vi "Spring Analysis.vi"() -> ()   [LabVIEW 2024]
uses:
  <vilib>/Utility/file.llb/Read Delimited Spreadsheet (DBL).vi
  <vilib>/gmath/NI_Gmath.lvlib
  <vilib>/Analysis/NI_AALPro.lvlib
panel:
  in  "Skip points (raw data)":i32
  out "Spectrum":T1(graph)=[{"time start"=0.0, "df"=0.49751243781094523, "Power Spectrum (V^2 rms)"=[5.644866949331598e-05, 0.00013686624305728217, 0.00022038571008669523, 0.00041028831547446017, 0.0008486507694054388, 0.002042096260864871, 0.006435671488207052, 0.020896992615224798, 0.010543505206445309, 0.00392758055394729, 0.001991571736893036, 0.0012169525544927543, 0.0008310812614828688, 0.0006098344085945337, 0.0004702652862590481, 0.000375985799513062, 0.0003089575120970624, 0.00025938177290646495, 0.00022154504395459433, 0.00019192243396481184, 0.00016823708014891692, 0.00014896115841386858, 0.00013303604254786888, 0.00011970786081307353, 0.00010842694010669756, 9.878417014082367e-05, 9.046951026584988e-05, 8.324421425577846e-05, 7.692180036901625e-05, 7.135474003886612e-05, 6.642497195524682e-05, 6.203702789756774e-05, 5.811297495461124e-05, 5.45886423520356e-05, 5.1410770806166024e-05, 4.853483372999109e-05, 4.5923354075646326e-05, 4.35445911853837e-05, 4.1371506917581324e-05, 3.938094472334656e-05, 3.7552972647060335e-05, 3.5870353631410695e-05, 3.431811550787647e-05, 3.288319965156931e-05, 3.155417216432179e-05, 3.032098510000748e-05, 2.917477799758377e-05, 2.8107712078341994e-05, 2.7112831065381034e-05, 2.6183943818827068e-05, 2.531552494024343e-05, 2.4502630250260028e-05, 2.3740824634033174e-05, 2.3026120216663534e-05, 2.235492320285061e-05, 2.1723988012796467e-05, 2.1130377585996665e-05, 2.0571428918158274e-05, 2.00447230537285e-05, 1.9548058884826993e-05, 1.9079430212451e-05, 1.8637005612268403e-05, 1.821911071872427e-05, 1.782421260036284e-05, 1.745090594850682e-05, 1.709790084256156e-05, 1.676401188963703e-05, 1.644814856514056e-05, 1.614930660539041e-05, 1.586656032393563e-05, 1.559905574077967e-05, 1.5346004428575323e-05, 1.5106677992571845e-05, 1.4880403111937629e-05, 1.4666557079393808e-05, 1.4464563784095495e-05, 1.4273890089585874e-05, 1.4094042564606332e-05, 1.392456452969376e-05, 1.3765033386971049e-05, 1.361505820442835e-05, 1.347427752938351e-05, 1.33423574087637e-05, 1.3218989596459617e-05, 1.3103889930277334e-05, 1.299679686299879e-05, 1.2897470133867677e-05, 1.2805689568343873e-05, 1.2721253995378978e-05, 1.2643980272694602e-05, 1.2573702411648248e-05, 1.2510270794245523e-05, 1.2453551475767183e-05, 1.2403425567259563e-05, 1.235978869287705e-05, 1.2322550517711422e-05, 1.2291634342378541e-05, 1.2266976761162613e-05, 1.224852738106678e-05, 1.2236248599588424e-05]}, {"time start"=0.0, "df"=0.5, "Power Spectrum (V^2 rms)"=[5.6303024605838505e-05, 0.00013698521619382454, 0.00022207111065130337, 0.0004162057648891435, 0.0008670327309824444, 0.002106953935671304, 0.006743647337272303, 0.02134435548843732, 0.010152944032489135, 0.003818664652887894, 0.0019521631638462402, 0.0011987461426457172, 0.000821227351523806, 0.0006039020886803867, 0.00046641372855931893, 0.00037334112300694406, 0.0003070617209886131, 0.00025797588434058424, 0.0002204735430536851, 0.00019108728072320526, 0.00016757393291649876, 0.00014842634075070798, 0.00013259904044947505, 0.00011934682035404783, 0.00010812586743173314, 9.853113532263249e-05, 9.02554633827969e-05, 8.306218604029104e-05, 7.676635083863324e-05, 7.122157081563383e-05, 6.63106489246679e-05, 6.193877966903397e-05, 5.802854430021882e-05, 5.451617525819134e-05, 5.134873261558307e-05, 4.8481945054995685e-05, 4.587854131814135e-05, 4.3506947970481254e-05, 4.1340263767530726e-05, 3.935544501430629e-05, 3.753265340009534e-05, 3.585473005500931e-05, 3.430676847514845e-05, 3.287576549051895e-05, 3.155033428420553e-05, 3.0320467084980642e-05, 2.9177337880358707e-05, 2.8113137568557535e-05, 2.7120935554807088e-05, 2.6194563022143593e-05, 2.5328514058508867e-05, 2.4517861566365142e-05, 2.375818546688881e-05, 2.3045511174664717e-05, 2.2376256688083065e-05, 2.1747186936257198e-05, 2.1155374261103743e-05, 2.059816410551022e-05, 2.0073145134689127e-05, 1.9578123145254e-05, 1.9111098220952924e-05, 1.8670244679907133e-05, 1.8253893429150234e-05, 1.7860516401094542e-05, 1.7488712795505423e-05, 1.713719689143336e-05, 1.680478722781218e-05, 1.6490396980207004e-05, 1.6193025385476953e-05, 1.5911750086642064e-05, 1.5645720287655987e-05, 1.5394150622599654e-05, 1.5156315656440666e-05, 1.4931544945310561e-05, 1.471921859351259e-05, 1.451876325243961e-05, 1.432964851343845e-05, 1.4151383652589758e-05, 1.3983514690501608e-05, 1.3825621734668978e-05, 1.3677316575829607e-05, 1.353824051312092e-05, 1.3408062385798106e-05, 1.3286476791860006e-05, 1.3173202476199866e-05, 1.3067980872899705e-05, 1.2970574788048847e-05, 1.2880767211031191e-05, 1.2798360243613115e-05, 1.2723174137392796e-05, 1.2655046431280431e-05, 1.2593831181663405e-05, 1.2539398278799699e-05, 1.249163284378996e-05, 1.2450434701207355e-05, 1.2415717923134284e-05, 1.2387410440970289e-05, 1.2365453721942524e-05, 1.234980250778595e-05, 1.2340424613557116e-05]}]
  out "w_n":dbl=22.360679774997898
  out "lambda":dbl=2.5
  out "phi":dbl=-6.379370208442803
  out "zeta":dbl=0.11180339887498948
  out "w":dbl=22.22048604328897
  in  "h (step rate)":dbl=0.01 format="%#_13g"
  in  "time end":dbl=2.0 format="%#_13g"
  out "formula":string="(1/0.2)*(0 - 100.0*x-1.0*v)"
  in  "b (kg/s)":dbl=1.0
  in  "k (N/m)":dbl=100.0
  in  "m (kg)":dbl=0.2
  out "XY Graph":cluster{"t":dbl[], "y":dbl[]}[](graph)=[{"t"=[0.0, 0.01, 0.02, 0.03, 0.04, 0.05, 0.06, 0.07, 0.08, 0.09, 0.1, 0.11, 0.12, 0.13, 0.14, 0.15, 0.16, 0.17, 0.18, 0.19, 0.2, 0.21, 0.22, 0.23, 0.24, 0.25, 0.26, 0.27, 0.28, 0.29, 0.3, 0.31, 0.32, 0.33, 0.34, 0.35000000000000003, 0.36, 0.37, 0.38, 0.39, 0.4, 0.41000000000000003, 0.42, 0.43, 0.44, 0.45, 0.46, 0.47000000000000003, 0.48, 0.49, 0.5, 0.51, 0.52, 0.53, 0.54, 0.55, 0.56, 0.5700000000000001, 0.58, 0.59, 0.6, 0.61, 0.62, 0.63, 0.64, 0.65, 0.66, 0.67, 0.68, 0.6900000000000001, 0.7000000000000001, 0.71, 0.72, 0.73, 0.74, 0.75, 0.76, 0.77, 0.78, 0.79, 0.8, 0.81, 0.8200000000000001, 0.8300000000000001, 0.84, 0.85, 0.86, 0.87, 0.88, 0.89, 0.9, 0.91, 0.92, 0.93, 0.9400000000000001, 0.9500000000000001, 0.96, 0.97, 0.98, 0.99, 1.0, 1.01, 1.02, 1.03, 1.04, 1.05, 1.06, 1.07, 1.08, 1.09, 1.1, 1.11, 1.12, 1.1300000000000001, 1.1400000000000001, 1.1500000000000001, 1.16, 1.17, 1.18, 1.19, 1.2, 1.21, 1.22, 1.23, 1.24, 1.25, 1.26, 1.27, 1.28, 1.29, 1.3, 1.31, 1.32, 1.33, 1.34, 1.35, 1.36, 1.37, 1.3800000000000001, 1.3900000000000001, 1.4000000000000001, 1.41, 1.42, 1.43, 1.44, 1.45, 1.46, 1.47, 1.48, 1.49, 1.5, 1.51, 1.52, 1.53, 1.54, 1.55, 1.56, 1.57, 1.58, 1.59, 1.6, 1.61, 1.62, 1.6300000000000001, 1.6400000000000001, 1.6500000000000001, 1.6600000000000001, 1.67, 1.68, 1.69, 1.7, 1.71, 1.72, 1.73, 1.74, 1.75, 1.76, 1.77, 1.78, 1.79, 1.8, 1.81, 1.82, 1.83, 1.84, 1.85, 1.86, 1.87, 1.8800000000000001, 1.8900000000000001, 1.9000000000000001, 1.9100000000000001, 1.92, 1.93, 1.94, 1.95, 1.96, 1.97, 1.98, 1.99, 2.0], "y"=[1.0, 0.975515625, 0.9048485799953885, 0.793683069664252, 0.6493929363281531, 0.4806011443268373, 0.29670008251256486, 0.10735789255481054, -0.07796451989619155, -0.2504628554170456, -0.40238498785058513, -0.5273561409768714, -0.6206213150931946, -0.6791972253554723, -0.7019307857362803, -0.6894658557932868, -0.6441243389898921, -0.569711583964797, -0.4712592311333951, -0.35472104410393157, -0.22663879090384154, -0.09379586235376258, 0.037123952080977934, 0.15985621065048394, 0.26883960656418304, 0.3594517673889705, 0.4281879550488793, 0.4727767722975505, 0.49223032830694485, 0.4868296232894181, 0.4580490211512866, 0.408426448734615, 0.3413882722918879, 0.26103956647665394, 0.1719316493186711, 0.07881928171138101, -0.01358017275140981, -0.10081402659302488, -0.1788976092955688, -0.2444849621427372, -0.29500018918659987, -0.32872500386549935, -0.34484035571892346, -0.34342235495225737, -0.3253949215470226, -0.292443568976384, -0.24689640504851432, -0.19157972789914587, -0.1296564691558737, -0.06445616690920357, 0.0006948609412173318, 0.06263490496802816, 0.11851238768904226, 0.16590922844963654, 0.20293713901309063, 0.22830349328088, 0.24134505591305894, 0.2420294992244689, 0.2309262055651196, 0.20914927105365919, 0.17827683439769085, 0.14025180322280553, 0.09726970640911173, 0.05165974680670299, 0.005765162700131027, -0.03817125792537532, -0.0781112015116528, -0.11230984961723836, -0.1393863044836639, -0.158372906037056, -0.16874207461187324, -0.1704104717672045, -0.16372138325677194, -0.1494072417839289, -0.1285350781827299, -0.10243838276656284, -0.07263934879204084, -0.04076574338519084, -0.008466705164658923, 0.022668389739429782, 0.0511842025707476, 0.07582357501558565, 0.09557891939612398, 0.10972898210465766, 0.1178599081398488, 0.11987034932104397, 0.1159611462422494, 0.10661083736652331, 0.09253887585301797, 0.07465893998148106, 0.054025087799386425, 0.03177372000252235, 0.009064374089703692, -0.012977717833028039, -0.03331460388033973, -0.05104176494358258, -0.0654255362421032, -0.07593040624916397, -0.08223536085077696, -0.08423901320416048, -0.08205381705083081, -0.07599017688950663, -0.06653171941364053, -0.05430335821716742, -0.04003405418447279, -0.024516338813351385, -0.008564724116440714, 0.007024926743547271, 0.021513141739166665, 0.03425000299447483, 0.04470234326186144, 0.05247394601235676, 0.05731810930030696, 0.05914233562598567, 0.05800530402270094, 0.0541066477962295, 0.04777038521758563, 0.039423117399039344, 0.02956830738133625, 0.018758080697674012, 0.007564037813668293, -0.0034514558511086115, -0.013762131287019213, -0.02290161425167547, -0.030483154208638476, -0.03621452415003514, -0.03990760318392188, -0.04148243580729574, -0.04096584007979952, -0.03848489812848742, -0.03425589469726605, -0.028569462935715474, -0.02177284379663645, -0.014250261390446144, -0.006402459262850092, 0.0013735676474944157, 0.008703670580218948, 0.015253603645054814, 0.02074331079027449, 0.024957884261405716, 0.02775482466611119, 0.02906743041485267, 0.028904340686160886, 0.02734544169485179, 0.0245345124303503, 0.020669126037913037, 0.01598843112513127, 0.010759509794696634, 0.005263044345776378, -0.00022097753341185095, -0.005426826720042466, -0.010115242655414573, -0.014083762428217628, -0.017174759029140417, -0.019280910109926268, -0.020347956959430813, -0.020374751853478153, -0.019410723717520652, -0.01755101108606643, -0.014929612490192732, -0.011710983614726916, -0.008080565062751212, -0.004234752905569823, -0.0003708262803258748, 0.003322676695688286, 0.006674689155693872, 0.00953907145920618, 0.011800492949357306, 0.01337853060978188, 0.014229872523405239, 0.014348611543999279, 0.013764708053206304, 0.012540785749171647, 0.010767497375390532, 0.008557755197001334, 0.006040161789274618, 0.0033519991759583434, 0.0006321383437194483, -0.001985782629107675, -0.004379593619351125, -0.006443966489134685, -0.008094709094618867, -0.009271823401027234, -0.0099412394552807, -0.010095205579256125, -0.009751381366060609, -0.008950740789438657, -0.007754445291027591, -0.006239888937871361, -0.004496148096187246, -0.0026190856517750516, -0.0007063643913824762, 0.0011473838458313055, 0.0028550062291457018, 0.004340696853274629, 0.005543124955016649, 0.0064177075783471696, 0.0069379580370410926, 0.007095889756472437, 0.006901501948259575, 0.006381416872882789]}, ...(2 in all)]
  # "Spring Mass Damper Model\n\nThis compares a Runga-Kutta solution to the analytical one.\n\nYou can add forcing if you want"
  # "Simulation parameters"
  # "Spring parameters"
  # "Calculated parameters"
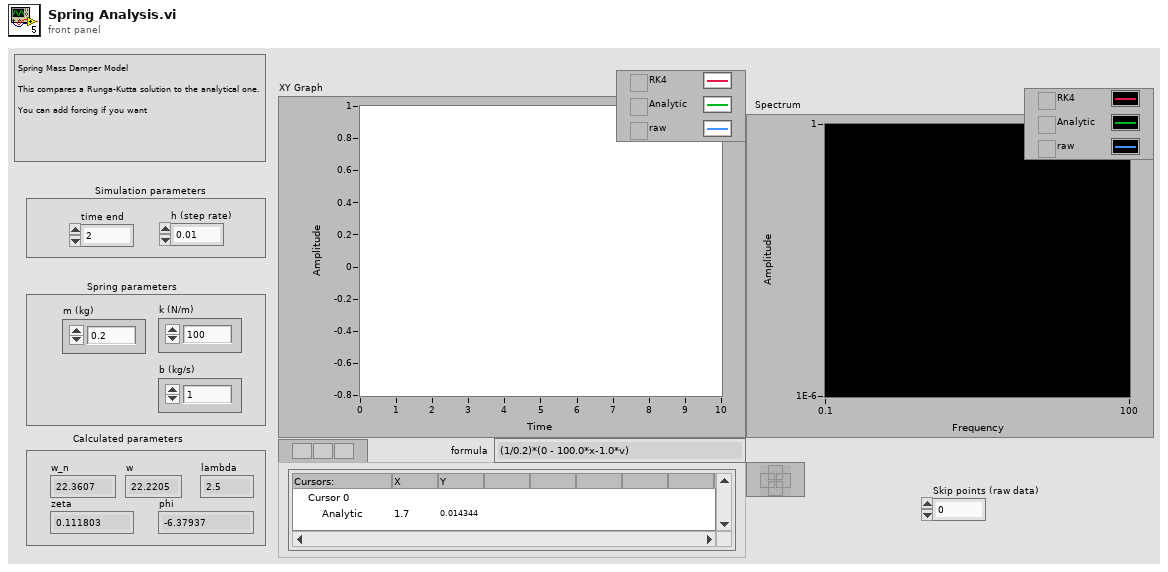
[diagram p1: front panel]
types:
  T1 = cluster{"time start":dbl, "df":dbl, "Power Spectrum (V^2 rms)":dbl[]}[]
  T2 = cluster{"time start":dbl, "df":dbl, "Power Spectrum (V^2 rms)":dbl[]}
  T3 = cluster{"Times":dbl[], "X Values (solution)":dbl[]}
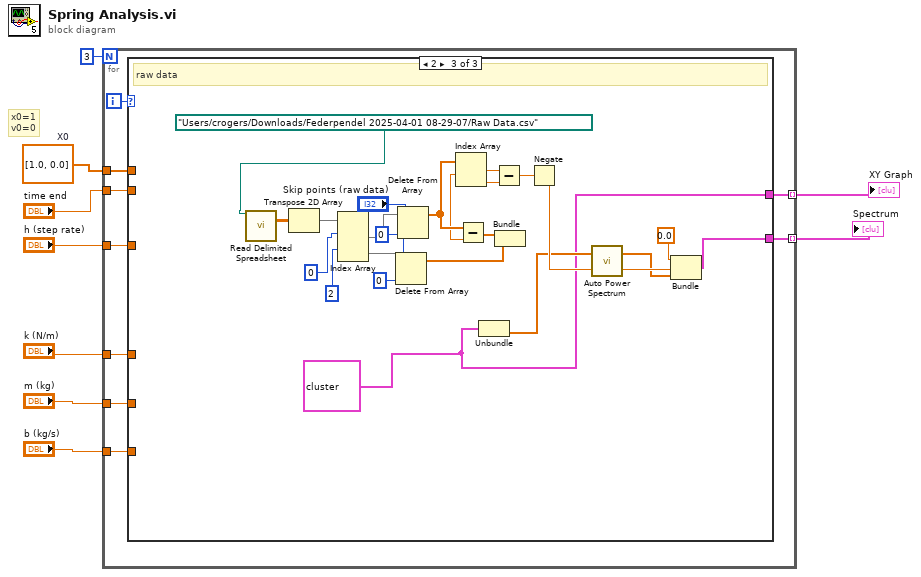
[diagram p0: block diagram]
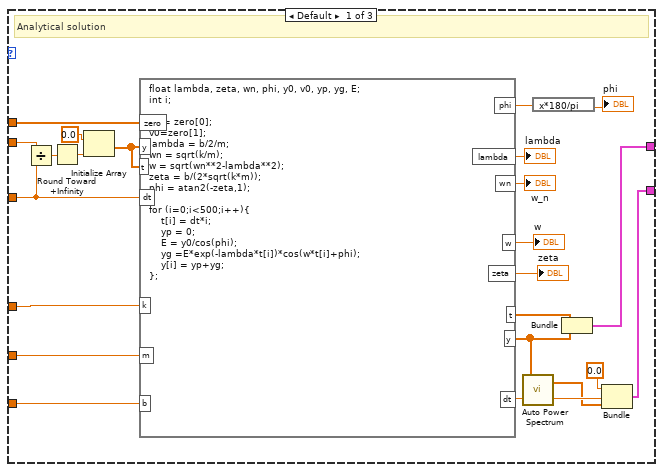
[diagram p2: hidden frame]
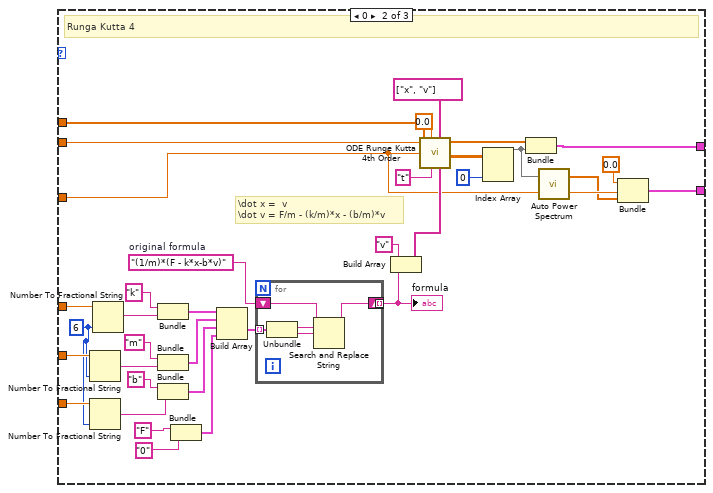
[diagram p3: hidden frame]
diagram:
  w5 = dbl[] [1.0, 0.0]  # X0
  # "x0=1\nv0=0"
  n1 = for {
    N: 3 -> [_]
    tunnel: "k (N/m)" -> [w18]
    tunnel: "m (kg)" -> [w17]
    tunnel: "b (kg/s)" -> [w16]
    tunnel: [w15] -> w4 mode=indexing
    tunnel: w5 -> [w14]
    tunnel: "h (step rate)" -> [w12]
    tunnel: "time end" -> [w11]
    tunnel: [w10] -> w1 mode=indexing
    i -> [w13]
    n2 = case shown="2" w13 {
      tunnel: w18 -> [w34 w61 _]
      tunnel: w17 -> [w33 w60 _]
      tunnel: w16 -> [w32 w59 _]
      tunnel: [w31 w58 w85] -> w15
      tunnel: w14 -> [w35 w57 _]
      tunnel: w12 -> [w29 w53 _]
      tunnel: w11 -> [w30 w56 _]
      tunnel: [w19 w49 w96] -> w10
      frame Default {
        # "Analytical solution"
        n3 = Divide(x=w30, y=w29) -> (x/y=w28:dbl)
        n4 = Round Toward +Infinity(x=w28) -> (ceil(x): smallest int >= x=w27:dbl)
        n5 = Initialize Array(0.0 ("element"), w27) -> (w39:dbl[])
        n6 = formula code="float lambda, zeta, wn, phi, y0, v0, yp, yg, E;\nint i;\n\ny0 = zero[0];\nv0=zero[1];\nlambda = b/2/m;\nwn = sqrt(k/m);\nw = sqrt(wn**2-lambda**2);\nzeta = b/(2*sqrt(k*m));\nphi = atan2(-zeta,1);\n\nfor (i=0;i<500;i++){\n    t[i] = dt*i;\n    yp = 0;\n    E = y0/cos(phi);\n    yg =E*exp(-lambda*t[i])*cos(w*t[i]+phi);\n    y[i] = yp+yg;\n};"("k"=w34, "m"=w33, "b"=w32, "dt"=w29, "y"=w39, "t"=w39, "zero"=w35) -> ("w"=→"w":dbl, "zeta"=→"zeta":dbl, "y"=w21:dbl[], "t"=w40:dbl[], "phi"=w41:dbl, "lambda"=→"lambda":dbl, "wn"=→"w_n":dbl, "dt"=w20:dbl)
        n7 = call <vilib>:"Auto Power Spectrum.vi"("dt"=w20, "Signal (V)"=w21) -> ("df"=w24:dbl, "Power Spectrum (V^2 rms)"=w23:dbl[])
        n8 = expression code="x*180/pi"(w41) -> (→"phi":dbl)
        n9 = Bundle("t"=w40, "y"=w21) -> (w31:cluster{"t":dbl[], "y":dbl[]})  [unwired: 1 in]
        n10 = Bundle("time start"=0.0, "df"=w24, "Power Spectrum (V^2 rms)"=w23) -> (w19:T2)  [unwired: 1 in]
      }
      frame 0 {
        w55 = i16 6 ("precision (6)")
        w45 = "(1/m)*(F - k*x-b*v)"  # original formula
        # "\\dot x =  v\n\\dot v = F/m - (k/m)*x - (b/m)*v"
        # "Runga Kutta 4"
        n11 = Number To Fractional String(number=w60, precision (6)=w55) -> (F-format string=w72:string)  [unwired: 2 out]
        n12 = Number To Fractional String(number=w59, precision (6)=w55) -> (F-format string=w66:string)  [unwired: 2 out]
        n13 = Number To Fractional String(number=w61, precision (6)=w55) -> (F-format string=w47:string)  [unwired: 2 out]
        n14 = Bundle("k", w47) -> (w68:cluster{string, string})  [unwired: 1 in]
        n15 = Bundle("m", w72) -> (w69:cluster{string, string})  [unwired: 1 in]
        n16 = Bundle("b", w66) -> (w67:cluster{string, string})  [unwired: 1 in]
        n17 = Bundle("F", "0") -> (w64:cluster{string, string})  [unwired: 1 in]
        n18 = Build Array(w68, w69, w67, w64) -> (w46:cluster{string, string}[])
        n19 = for {
          tunnel: w46 -> [w83] mode=indexing
          shift-right: [w79] -> w44
          shift-left: w45 -> [w82]
          tunnel: [w79] -> _ mode=indexing
          n20 = Unbundle(w83) -> (w81:string, w80:string)
          n21 = Search and Replace String(input string=w82, search string=w81, replace string=w80) -> (result string=w79:string)  [unwired: 5 in, 3 out]
        }
        "formula" <- w44
        n22 = Build Array("v", w44) -> (w62:string[])
        n23 = call <vilib>:"ODE Runge Kutta 4th Order.vi"("time end"=w56, "time start"=0.0, "h (step rate)"=w53, "X0"=w57, "time"="t", "X (name of variables)"=string[] ["x", "v"], "F(X,t) (right sides of the ODE\nas functions of X and t)"=w62) -> ("Times"=w75:dbl[], "X Values (solution)"=w73:dbl[][])  [unwired: 2 out]
        n24 = Index Array(array=w73, index (col)=0) -> (element=w54:dbl[])  [unwired: 1 in]
        n25 = Bundle("Times"=w75, "X Values (solution)"=w54) -> (w58:T3)  [unwired: 1 in]
        n26 = call <vilib>:"Auto Power Spectrum.vi"("dt"=w53, "Signal (V)"=w54) -> ("df"=w52:dbl, "Power Spectrum (V^2 rms)"=w51:dbl[])
        n27 = Bundle("time start"=0.0, "df"=w52, "Power Spectrum (V^2 rms)"=w51) -> (w49:T2)  [unwired: 1 in]
      }
      frame 2 {
        w85 = cluster{"all rows":dbl[], "all rows":dbl[]} {"all rows"=array[947 elements], "all rows"=array[947 elements]} ("XY Graph")
        # "raw data"
        n28 = call-poly <vilib>:"Read Delimited Spreadsheet.vi"("file path (dialog if empty)"=path "/Users/crogers/Downloads/Federpendel 2025-04-01 08-29-07/Raw Data.csv") -> ("all rows"=w106:dbl[][])  [unwired: 9 in, 5 out]
        n29 = Transpose 2D Array(2D array=w106) -> (transposed array=w95:dbl[][])
        n30 = Index Array(array=w95, index (row) #1=0 ("index (row)"), index (row) #2=2 ("index (row)")) -> (element #1=w100:dbl[], element #2=w92:dbl[])  [unwired: 2 in]
        n31 = Delete From Array(array=w92, length="Skip points (raw data)", index=0) -> (array with subset deleted=w87:dbl[])  [unwired: 1 out]
        n32 = Delete From Array(array=w100, length="Skip points (raw data)", index=0) -> (array with subset deleted=w91:dbl[])  [unwired: 1 out]
        n33 = Index Array(array=w91) -> (element #1=w90:dbl, element #2=w99:dbl)  [unwired: 2 in]
        n34 = Subtract(x=w91, y=w90) -> (x-y=w89:dbl[])
        n35 = Unbundle(w85) -> ("all rows"=w86:dbl[])  [unwired: 1 out]
        n36 = Subtract(x=w90, y=w99) -> (x-y=w98:dbl)
        n37 = Bundle(w89, w87) -> ()  [unwired: 1 in, 1 out]
        n38 = Negate(x=w98) -> (-x=w97:dbl)
        n39 = call <vilib>:"Auto Power Spectrum.vi"("dt"=w97, "Signal (V)"=w86) -> ("df"=w103:dbl, "Power Spectrum (V^2 rms)"=w102:dbl[])
        n40 = Bundle("time start"=0.0, "df"=w103, "Power Spectrum (V^2 rms)"=w102) -> (w96:T2)  [unwired: 1 in]
      }
    }
  }
  "XY Graph" <- w4
  "Spectrum" <- w1
